vi "State Machine.vi"   [LabVIEW 2020, in "State Machine.lvlib"]
uses:
  State Machine.lvlib
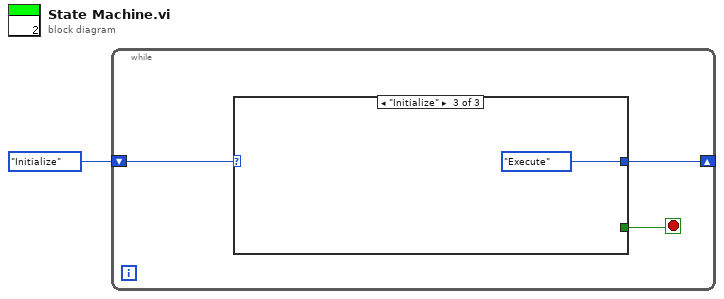
[diagram p0: block diagram]
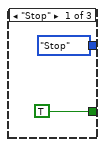
[diagram p2: hidden frame]
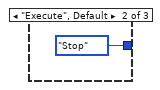
[diagram p3: hidden frame]
diagram:
  n1 = while {
    shift-right: [w3] -> _
    shift-left: enum16{"Stop", "Execute", "Initialize"}."Initialize" -> [w4]
    stop <- w2 stop-if-true
    n2 = case shown="\"Initialize\"" w4 {
      tunnel: [enum16{"Stop", "Execute", "Initialize"}."Stop" enum16{"Stop", "Execute", "Initialize"}."Stop" enum16{"Stop", "Execute", "Initialize"}."Execute"] -> w3
      tunnel: [TRUE _ _] -> w2
      frame "Stop" {
      }
      frame "Execute", Default {
      }
      frame "Initialize" {
      }
    }
  }
